vi "setMagnetVector.vi"(8 "error in (no error)":errorcluster, 9 "Target Rate (T/min)":dbl, 10 "Target Field (T)":dbl[](array[numeric]), 11 "Instrument.Cryostat in":refnum<class "Instrument.Cryostat.lvclass">) -> (0 "error out":errorcluster, 3 "Instrument.Cryostat out":refnum<class "Instrument.Cryostat.lvclass">)   [LabVIEW 2019, in "Instrument.Cryostat.lvclass"]
uses:
  Instrument.Cryostat.lvclass
  Typedefs/setMagnetVector--cluster.ctl
  Typedefs/Cryostat.commands--enum.ctl
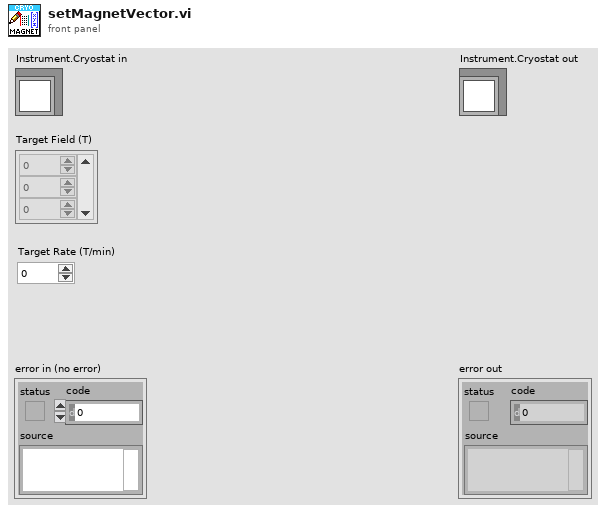
[diagram p1: front panel]
types:
  T1 = typedef "Instrument.Cryostat.lvclass/Cryostat.commands--enum.ctl" = enum16{"getLN2Level", "getLHeLevel", "getMagnet", "getMagnetVector", "setMagnet", "setMagnetVector", "getAngle", "setAngle", "getTemperature", "setTemperature", "getHeater", "setHeater", "getChamber", "setChamber", "getPressure"}
  T2 = typedef "Instrument.Cryostat.lvclass/setMagnetVector--cluster.ctl" = cluster{"field":dbl[], "rate":dbl}
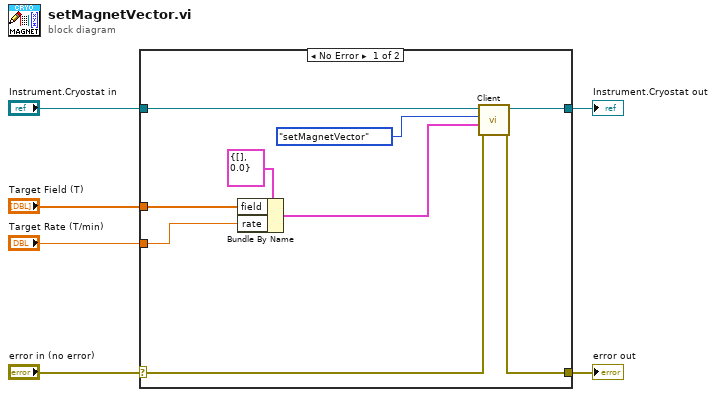
[diagram p0: block diagram]
diagram:
  n1 = case shown="No Error" "error in (no error)" {
    selector: "error in (no error)" -> [w7 w17]
    tunnel: [w13 w17] -> w5
    tunnel: [w11 w16] -> w3
    tunnel: "Instrument.Cryostat in" -> [w8 w16]
    tunnel: "Target Field (T)" -> [w15 _]
    tunnel: "Target Rate (T/min)" -> [w14 _]
    frame No Error {
      n2 = Bundle By Name(cluster=T2 {"field"=[], "rate"=0.0} ("setMagnet"), "field"=w15, "rate"=w14) -> (w12:T2)
      n3 = call-dynamic "Client.vi"("error in (no error)"=w7, "Data in"=w12, "Command in"=Cryostat.commands--enum."setMagnetVector" ("commands"), "Instrument in"=w8) -> ("error out"=w13:errorcluster, "Instrument out"=w11:refnum<class "Instrument.Cryostat.lvclass">)  [unwired: 4 in, 2 out]
    }
    frame Error {
    }
  }
  "error out" <- w5
  "Instrument.Cryostat out" <- w3
